vi "calculo tração do subvão a HT.vi"() -> ()   [LabVIEW 2020]
panel:
  out "T01ht":dbl
  out "To2 Real  (N)":dbl=17749.49999999993 format="%.3f"
  in  "S cond (m²)":dbl=0.0005168
  in  "E cond (Pa)":dbl=65500000000.0
  in  "Alfa t (1/°C)":dbl=2.09e-05
  in  "t2-t1 (°C)":dbl=35.0
  out "fsub cond 02":dbl
  out "L":dbl
  out "f EDS cond 2":dbl
  in  "p cond":dbl
  in  "Ext.lim (m)":dbl
  in  "Tração EDS cond":dbl
  out "A sub ht":dbl
  out "Var A sup":dbl
  in  "E sup":dbl
  in  "S sup":dbl
  in  "Var T0sup":dbl
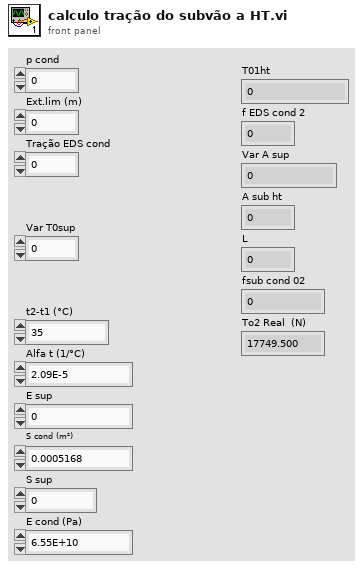
[diagram p1: front panel]
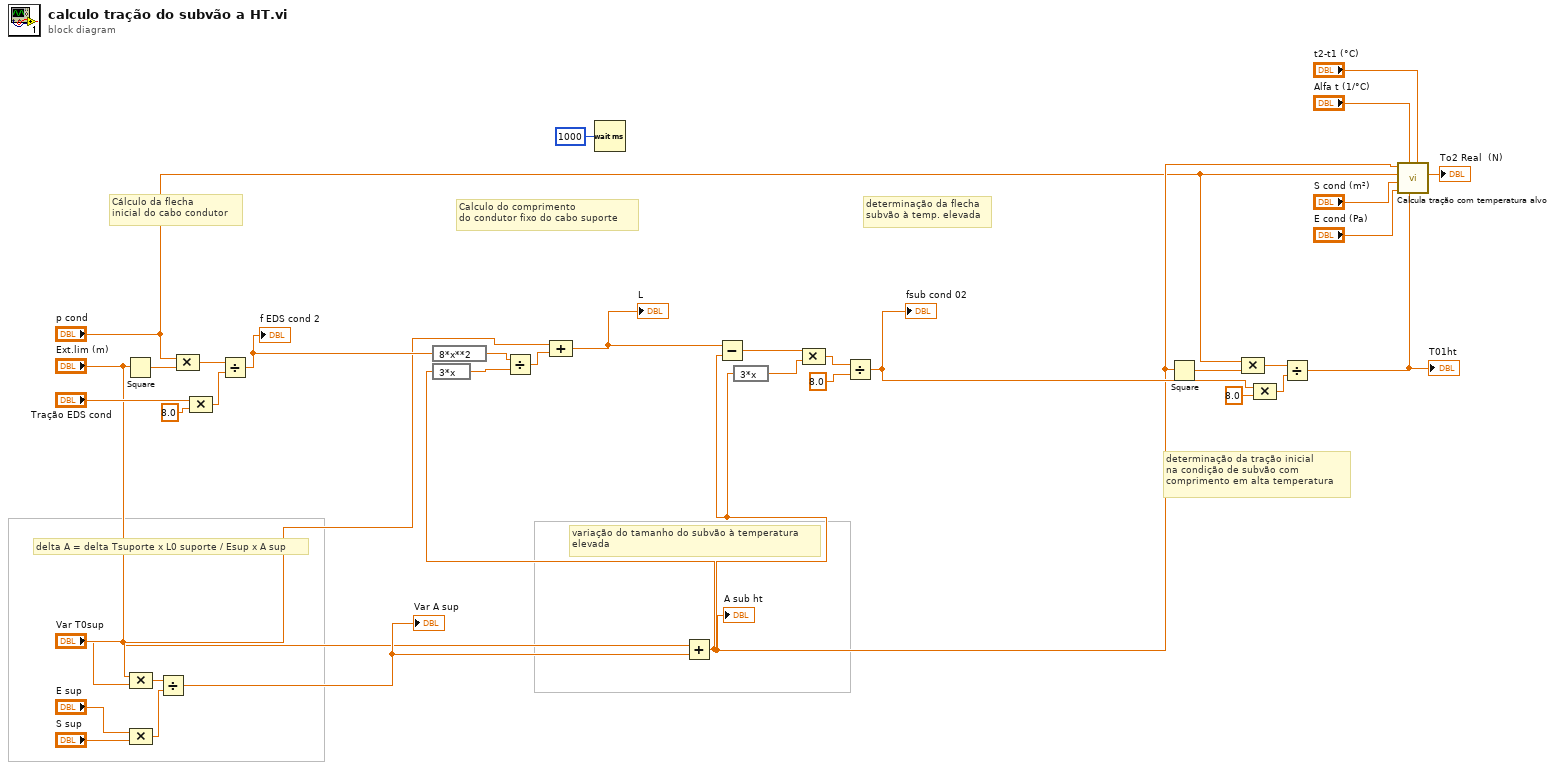
[diagram p0: block diagram]
diagram:
  # "determinação da tração inicial \nna condição de subvão com \ncomprimento em alta temperatura"
  # "determinação da flecha\nsubvão à temp. elevada"
  # "Calculo do comprimento\ndo condutor fixo do cabo suporte"
  # "Cálculo da flecha\ninicial do cabo condutor"
  # "variação do tamanho do subvão à temperatura\nelevada"
  # "delta A = delta Tsuporte x L0 suporte / Esup x A sup"
  n1 = Square(x="Ext.lim (m)") -> (x^2=w25:dbl)
  n2 = Compound Arithmetic op=MULTIPLY("Var T0sup", "Ext.lim (m)") -> (w34:dbl)
  n3 = Compound Arithmetic op=MULTIPLY("E sup", "S sup") -> (w31:dbl)
  n4 = Divide(x=w34, y=w31) -> (x/y=w30:dbl)
  "Var A sup" <- w30
  n5 = Compound Arithmetic op=MULTIPLY("p cond", w25) -> (w27:dbl)
  n6 = Compound Arithmetic op=MULTIPLY("Tração EDS cond", 8.0 ("value")) -> (w29:dbl)
  n7 = Divide(x=w27, y=w29) -> (x/y=w24:dbl)
  "f EDS cond 2" <- w24
  n8 = expression code="8*x**2"(w24) -> (w22:dbl)
  n9 = Wait (ms)(milliseconds to wait=u32 1000) -> ()  [unwired: 1 out]
  n10 = Add(x="Ext.lim (m)", y=w30) -> (x+y=w5:dbl)
  "A sub ht" <- w5
  n11 = expression code="3*x"(w5) -> (w21:dbl)
  n12 = Divide(x=w22, y=w21) -> (x/y=w23:dbl)
  n13 = Compound Arithmetic op=ADD("Ext.lim (m)", w23) -> (w20:dbl)
  "L" <- w20
  n14 = Subtract(x=w20, y=w5) -> (x-y=w19:dbl)
  n15 = expression code="3*x"(w5) -> (w16:dbl)
  n16 = Compound Arithmetic op=MULTIPLY(w19, w16) -> (w18:dbl)
  n17 = Divide(x=w18, y=8.0) -> (x/y=w13:dbl)
  "fsub cond 02" <- w13
  n18 = Square(x=w5) -> (x^2=w2:dbl)
  n19 = Compound Arithmetic op=MULTIPLY("p cond", w2) -> (w14:dbl)
  n20 = Compound Arithmetic op=MULTIPLY(w13, 8.0 ("value")) -> (w15:dbl)
  n21 = Divide(x=w14, y=w15) -> (x/y=w11:dbl)
  "T01ht" <- w11
  n22 = call "Calcula tração com temperatura alvo.vi"("t2-t1 (°C)"="t2-t1 (°C)", "To1 (N)"=w11, "Alfa t (1/°C)"="Alfa t (1/°C)", "E (Pa)"="E cond (Pa)", "S (m²)"="S cond (m²)", "p (N/m)"="p cond", "Ao (m)"=w5) -> ("To2 Real  (N)"=→"To2 Real  (N)":dbl)  [unwired: 4 in]
